vi "MacroTiming_Update.vi"(8 "error in (no error)":errorcluster, 10 "UI control refnums":T1, 11 "Macro Error IN?":bool) -> (0 "error out":errorcluster)   [LabVIEW 2012]
doc: "SciScan 1.2 160622"
uses:
  Custom Controls and Typedefs/Macro_MD_UI Control Refnums.ctl
  Custom Controls and Typedefs/Delete Button.ctl
  Custom Controls and Typedefs/Edit Button.ctl
  Custom Controls and Typedefs/Timing Estimate Cluster.ctl
  CommonResource VIs/Timing/Timing Indicator.ctl
  Custom Controls and Typedefs/Load from PSM Button.ctl
panel:
  # "(hh:mm:ss)"
  # "(hh:mm:ss)"
  # "(hh:mm:ss)"
  # "(hh:mm:ss)"
  # "(hh:mm:ss)"
  # "(hh:mm:ss)"
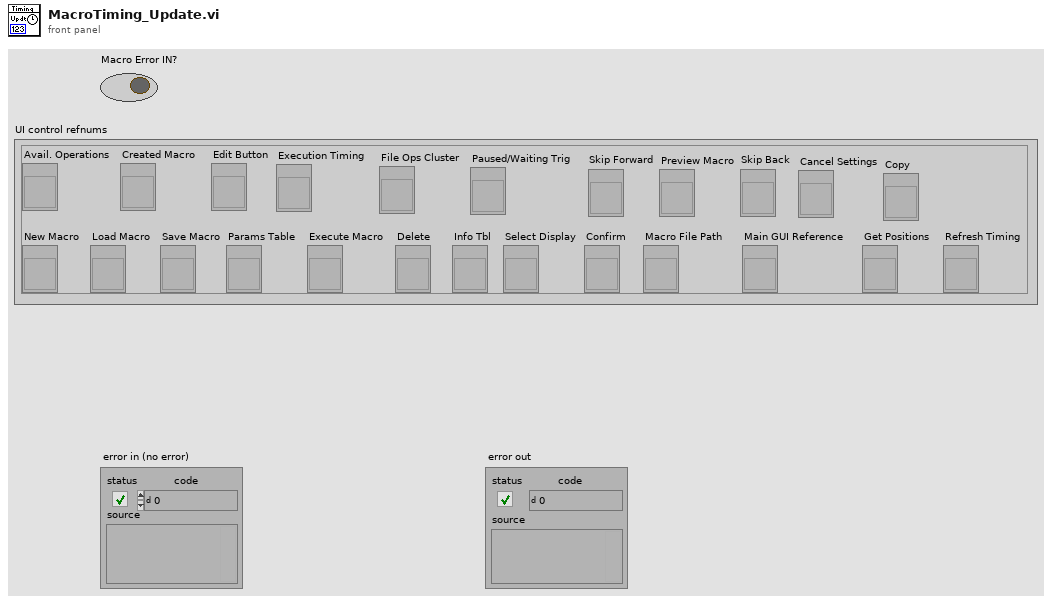
[diagram p1: front panel]
types:
  T1 = typedef "Macro_MD_UI Control Refnums.ctl" = cluster{"Avail. Operations":refnum<vi>, "Created Macro":refnum<vi>, "Load Macro":refnum<vi>, "Save Macro":refnum<vi>, "Params Table":refnum<vi>, "Delete":refnum<vi>, "Edit Button":refnum<vi>, "Execute Macro":refnum<vi>, "Info Tbl":refnum<vi>, "Execution Timing":refnum<vi>, "Select Display":refnum<vi>, "File Ops Cluster":refnum<vi>, "Paused/Waiting Trig":refnum<vi>, "Confirm":refnum<vi>, "New Macro":refnum<vi>, "Preview Macro":refnum<vi>, "Skip Forward":refnum<vi>, "Skip Back":refnum<vi>, "Macro File Path":refnum<vi>, "Main GUI Reference":refnum<vi>, "Cancel Settings":refnum<vi>, "Get Positions":refnum<vi>, "Copy":refnum<vi>, "Refresh Timing":refnum<vi>}
  T2 = typedef "Timing Estimate Cluster.ctl" = cluster{"Est. Time":dbl, "Remaining":dbl, "Progress":u8, "Elapsed":dbl}
  T3 = cluster{"Estimated Run time":dbl, "Step by step exec time":dbl[]}
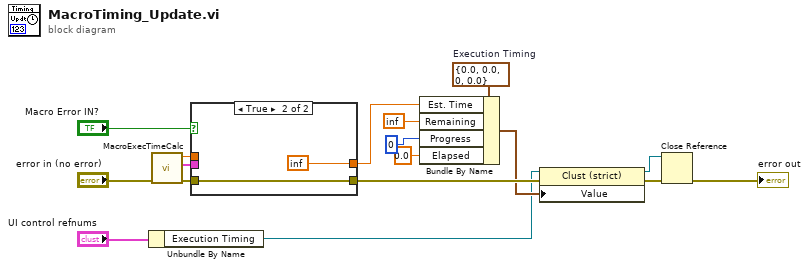
[diagram p0: block diagram]
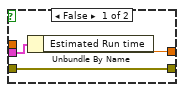
[diagram p2: hidden frame]
diagram:
  w8 = T2 {"Est. Time"=0.0, "Remaining"=0.0, "Progress"=0, "Elapsed"=0.0}  # Execution Timing
  n1 = Unbundle By Name("UI control refnums") -> ("Execution Timing"=w2:refnum<vi>)
  n2 = call "MacroExecTimeCalc.vi"("Error In"="error in (no error)") -> ("Error Out"=w16:errorcluster, "Estimated Timing cluster"=w14:T3, "Estimated Time"=w17:dbl)  [unwired: 8 in]
  n3 = case shown="True" "Macro Error IN?" {
    tunnel: w17 -> [_ _]
    tunnel: w16 -> [w20 w21]
    tunnel: [w18 inf] -> w15
    tunnel: [w20 w21] -> w13
    tunnel: w14 -> [w19 _]
    frame False {
      n4 = Unbundle By Name(w19) -> ("Estimated Run time"=w18:dbl)
    }
    frame True {
    }
  }
  n5 = Bundle By Name(cluster=w8, "Est. Time"=w15, "Remaining"=inf, "Progress"=u8 0, "Elapsed"=0.0) -> (w10:T2)
  n6 = property class="Clust (strict)"(reference=w2, error in=w13, "Value"=w10) -> (reference out=w6:refnum<vi>, error out=w7:errorcluster)
  n7 = Close Reference(reference=w6, error in (no error)=w7) -> (error out=→"error out":errorcluster)
